vi "停止.vi"(8 "error in (no error)":errorcluster caption="错误输入（无错误）", 11 "生命游戏 输入":refnum<class "生命游戏.lvclass">) -> (0 "error out":errorcluster caption="错误输出", 3 "生命游戏 输出":refnum<class "生命游戏.lvclass">)   [LabVIEW 2015, in "生命游戏.lvlib" / "生命游戏.lvclass"]
uses:
  <vilib>/ActorFramework/Time-Delayed Send Message/Time-Delay Override Options.ctl
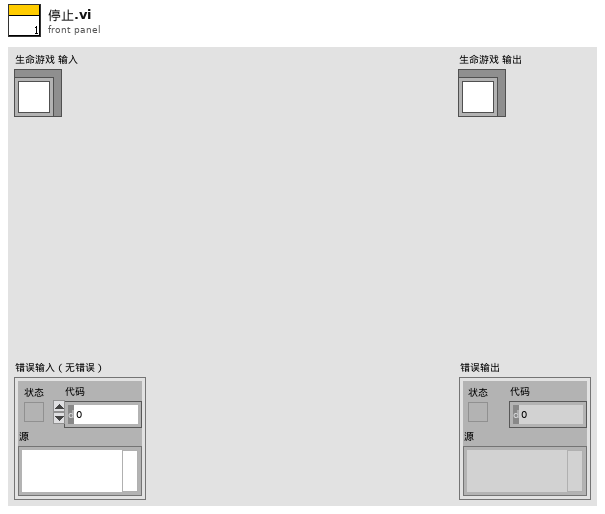
[diagram p1: front panel]
types:
  T1 = typedef "Time-Delay Override Options.ctl" = enum16{"Send next copy now", "Skip next scheduled copy", "Send next copy now and stop all further copies", "Stop all further copies"}
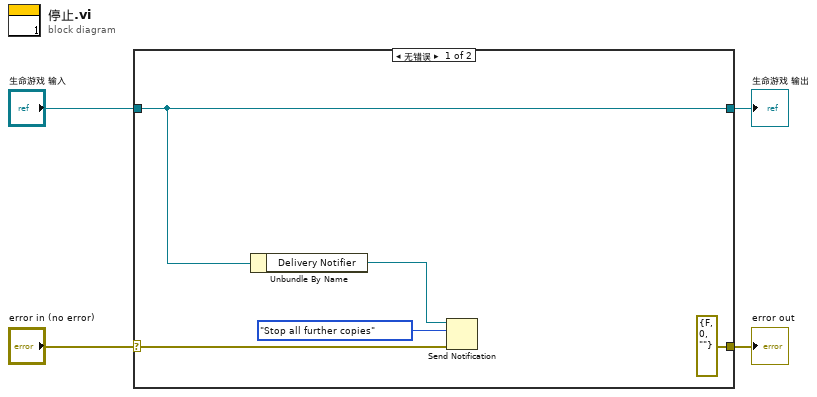
[diagram p0: block diagram]
diagram:
  n1 = case shown="无错误" "error in (no error)" {
    selector: "error in (no error)" -> [w6 w11]
    tunnel: [errorcluster {"status"=FALSE, "code"=0, "source"=""} ("error IO") w11] -> w3
    tunnel: [w9 w10] -> w1
    tunnel: "生命游戏 输入" -> [w9 w10]
    frame No Error {
      n2 = Unbundle By Name(w9) -> ("Delivery Notifier"=w8:refnum<notifier>)
      n3 = Send Notification(notification=Time-Delay_Override_Options."Stop all further copies" ("通知"), notifier=w8, error in (no error)=w6) -> ()  [unwired: 2 out]
    }
    frame Error {
    }
  }
  "error out" <- w3
  "生命游戏 输出" <- w1
